vi "Download_Latest_Build.vi"(0 "Save Path":path=path "C:/Automation/APLs", 5 "Artifactory Program Name":string="avenger_rc17", 11 "Error In":errorcluster) -> (4 "Output Path":path, 6 "Output Path String":string, 15 "Error Out":errorcluster)   [LabVIEW 2016]
uses:
  <vilib>/regexp/Match Regular Expression.xnode
  <vilib>/httpClient/LabVIEWHTTPClient.lvlib
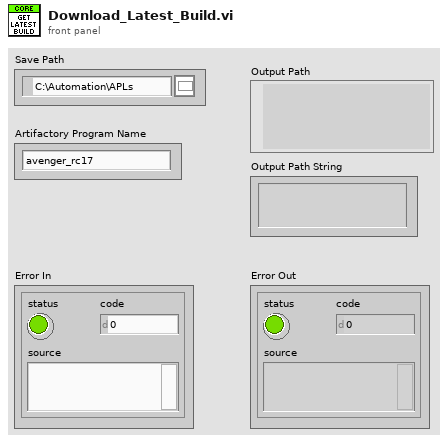
[diagram p1: front panel]
types:
  T1 = typedef "LabVIEWHTTPClient.lvlib/ClientHandle.ctl" = refnum<k1>
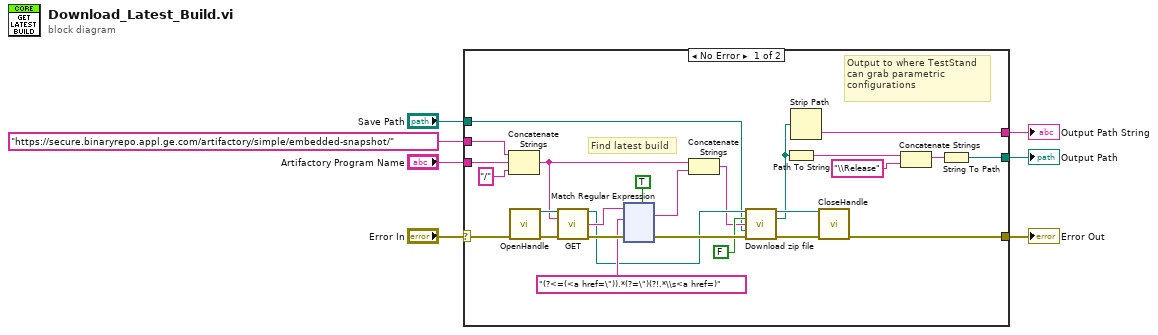
[diagram p0: block diagram]
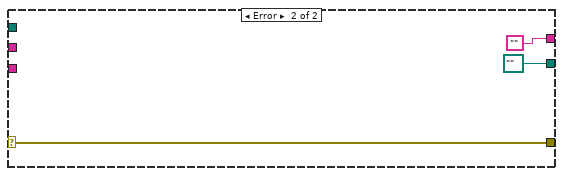
[diagram p2: hidden frame]
diagram:
  n1 = case shown="No Error" "Error In" {
    selector: "Error In" -> [w31 w150]
    tunnel: [w16 w150] -> w6
    tunnel: [w20 path ""] -> w2
    tunnel: "Artifactory Program Name" -> [w25 _]
    tunnel: "https://secure.binaryrepo.appl.ge.com/artifactory/simple/embedded-snapshot/" ("regular expression") -> [w26 _]
    tunnel: "Save Path" -> [w12 _]
    tunnel: [w8 ""] -> w1
    frame No Error {
      # "Output to where TestStand\ncan grab parametric\nconfigurations"
      # "Find latest build"
      n2 = Concatenate Strings(w26, w25, "/" ("string")) -> (w27:string)
      n3 = call <vilib>:"OpenHandle.vi"("error in (no error)"=w31) -> ("client handle out"=w32:T1, "error out"=w33:errorcluster)  [unwired: 13 in]
      n4 = call <vilib>:"GET.vi"("client handle"=w32, "url"=w27, "error in (no error)"=w33) -> ("client handle out"=w15:T1, "body"=w29:string, "error out"=w30:errorcluster)  [unwired: 9 in, 1 out]
      n5 = xnode "Match Regular Expression"("input string"=w29, "regular expression"="(?<=(<a href=\")).*(?=\")(?!.*\\s<a href=)", "error in"=w30, "multiline? (F)"=TRUE) -> ("whole match"=w28:string, "error out"=w18:errorcluster)  [unwired: 2 in, 3 out]
      n6 = Concatenate Strings(w27, w28) -> (w13:string)
      n7 = call "Download zip file.vi"("client handle"=w15, "Standalone?"=FALSE, "Artifactory ZIP Directory"=w13, "Save Path"=w12, "Error In"=w18) -> ("client handle out"=w11:T1, "Output Path"=w10:path, "Error Out"=w17:errorcluster)  [unwired: 8 in]
      n8 = Path To String(path=w10) -> (string=w9:string)
      n9 = Strip Path(path=w10) -> (name=w8:string)  [unwired: 1 out]
      n10 = call <vilib>:"CloseHandle.vi"("client handle"=w11, "error in (no error)"=w17) -> ("error out"=w16:errorcluster)  [unwired: 13 in]
      n11 = Concatenate Strings(w9, "\\Release" ("string")) -> (w19:string)
      n12 = String To Path(string=w19) -> (path=w20:path)
    }
    frame Error {
    }
  }
  "Error Out" <- w6
  "Output Path" <- w2
  "Output Path String" <- w1
